vi "ziGetValueDouble.vi"(3 "error in":errorcluster, 4 "Path":string, 5 "Handle in":T1 {"Handle" format="0x%08x"; "Conn" format="0x%08x"}) -> (0 "error out":errorcluster, 1 "Value":dbl, 2 "Handle out":T1 {"Handle" format="0x%08x"; "Conn" format="0x%08x"})   [LabVIEW 2016, in "Zurich Instruments LabOne.lvlib"]
doc: "This vi retrieves the numerical value of the specified node as an double-type value. The vi returns the value first found that matches Path if more than one value is available (a wildcard is used in the Path)."
uses:
  Zurich Instruments LabOne.lvlib
  ziTypeHandle.ctl
  Private/ziLV64.framework
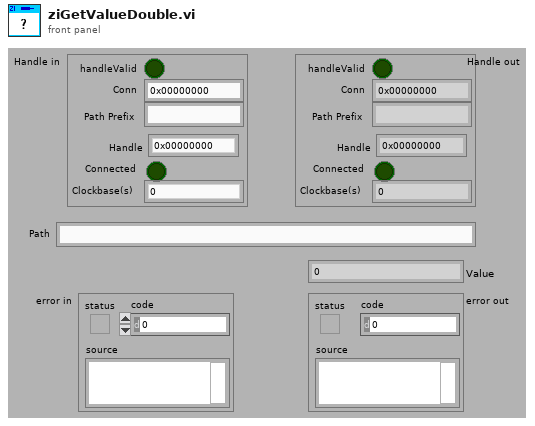
[diagram p1: front panel]
types:
  T1 = typedef "Zurich Instruments LabOne.lvlib/ziTypeHandle.ctl" = cluster{"handleValid":bool, "Conn":u64, "Path Prefix":string, "Handle":u64, "Connected":bool, "Clockbase(s)":dbl}
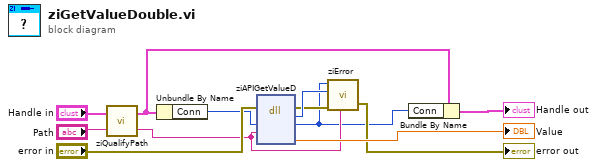
[diagram p0: block diagram]
diagram:
  n1 = call "ziQualifyPath.vi"("Path In"="Path", "Handle In"="Handle in") -> ("Path Out"=w2:string, "Handle Out"=w3:T1)
  n2 = Unbundle By Name(w3) -> ("Conn"=w11:u64)
  n3 = dll-call lib="Users/arkady/Desktop/ado/github/resonant_ultrasound_arxiv/maglab ultrasound -- arkady --arxiv/Zurich/Zurich Instruments/LabOne/API/LabVIEW/Zurich Instruments LabOne/Private/ziLV*.*" fn="ziAPIGetValueD"(error in="error in", "Conn"=w11, "Path"=w2) -> (error out=w8:errorcluster, "return type"=w9:u32, "Conn"=w1:u64, "Value"=→"Value":dbl)  [unwired: 2 in, 3 out]
  n4 = call "ziError.vi"("Conn"=w1, "ziErrorCode"=w9, "Error In"=w8, "Annotation"=w2) -> ("Error Out"=→"error out":errorcluster)  [unwired: 1 in, 1 out]
  n5 = Bundle By Name(cluster=w3, "Conn"=w1) -> (→"Handle out":T1)
